vi "PH_StatusHandler.constructor.vi"(0 "name":string, 2 "data in":string, 5 "error in(no error)":errorcluster) -> (14 "i ref out":refnum<vi>, 16 "data out":string, 19 "error out":errorcluster)   [LabVIEW 2014, in "PH_StatusHandler.lvlib"]
doc: "This class is forseen to control black boxes (motion).\n\nThis class is part of the PHELIX device layer.\n\nauthor: Stefan Götte, GSI\n\nLicense Agreement for this software:\n\nCopyright (C)\nGesellschaft für Schwerionenforschung, GSI\nPlanckstr. 1\n64291 Darmstadt\nGermany\n\nContact: D.Beck@gsi.de \n\nThis program is free software; you can redistribute it and/or modify it under the terms of the \nGNU General Public License as published by the Free Software Foundation; either version 2 of \nthe license, or (at your option) any later version.\n\nThis program is distributed in the hope that it will be useful, but WITHOUT ANY WARRANTY; \nwithout even the implied warranty of MERCHANTABILITY or FITNESS FOR A PARTICULAR PURPOSE. See the GNU General License for more details (http://www.gnu.org).\n\nGesellschaft für Schwerionenforschung, GSI\nPlanckstr. 1, 64291 Darmstadt, Germany\nFor all questions and ideas contact: M.Richter@gsi.de, H.Brand@gsi.de or D.Beck@gsi.de.\nLast update: 16-JUN-2004"
uses:
  PH_StatusHandler.lvlib
  CS_Core/CSSystem/CSSystemLib/CSSystemLib.lvlib
  PH_Class/PH_Class.lvlib
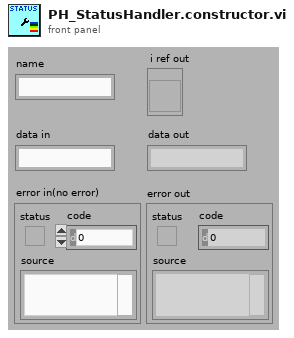
[diagram p1: front panel]
types:
  T1 = enum16{"SetAttribute", "GetAttribute", "CreateAttribute", "DestroyAttribute", "DestroyAllAtributes"}
  T2 = typedef "PH_StatusHandler.lvlib/PH_StatusHandler.i attribute.ctl" = cluster{"GUI Ref":refnum<vi>, "Value":T3, "Service ID":i32}
  T3 = typedef "PH_StatusHandler.lvlib/PH_StatusHandler.Status.ctl" = i16
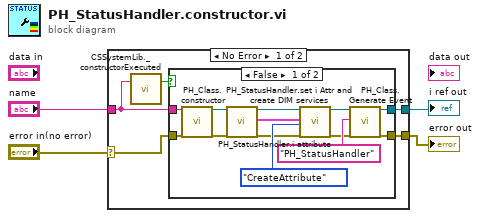
[diagram p0: block diagram]
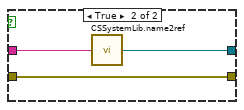
[diagram p2: hidden frame]
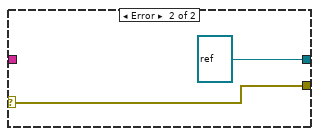
[diagram p3: hidden frame]
diagram:
  n1 = case shown="No Error" "error in(no error)" {
    selector: "error in(no error)" -> [w9 w27]
    tunnel: [w7 refnum<vi> refnum ("i ref out")] -> w4
    tunnel: [w8 w27] -> w3
    tunnel: "name" -> [w6 _]
    frame No Error {
      n2 = call "CSSystemLib._constructorExecuted.vi"("name"=w6) -> ("constructor executed?"=w5:bool)  [unwired: 18 in]
      n3 = case shown="False" w5 {
        tunnel: w9 -> [w16 w25]
        tunnel: [w14 w25] -> w8
        tunnel: [w15 w23] -> w7
        tunnel: w6 -> [w21 w24]
        frame False {
          n4 = call "PH_Class.constructor.vi"("name"=w21, "error in"=w16) -> ("i ref out"=w12:refnum<vi>, "error out"=w19:errorcluster)  [unwired: 15 in, 1 out]
          n5 = call "PH_StatusHandler.set i Attr and create DIM services.vi"("VI in"=w12, "error in (no error)"=w19) -> ("VI out"=w11:refnum<vi>, "i attribute"=w10:T2, "error out"=w13:errorcluster)  [unwired: 15 in]
          n6 = call "PH_StatusHandler.i attribute.vi"("VI Refnum"=w11, "CLASS.i attribute"=w10, "Action"=T1."CreateAttribute", "error in (no error)"=w13) -> ("VI Refnum out"=w18:refnum<vi>, "error out"=w17:errorcluster)  [unwired: 13 in, 1 out]
          n7 = call "PH_Class.Generate Event.vi"("i ref in"=w18, "Class"="PH_StatusHandler", "error in (no error)"=w17) -> ("i ref out"=w15:refnum<vi>, "error out"=w14:errorcluster)  [unwired: 15 in]
        }
        frame True {
          n8 = call "CSSystemLib.name2ref.vi"("name"=w24) -> ("obj refnum"=w23:refnum<vi>)
        }
      }
    }
    frame Error {
    }
  }
  "i ref out" <- w4
  "error out" <- w3
